vi "DriveStraightCommandNavXRamparts.vi"(6 "TONDelay":u32=50, 8 "speed":dbl=0.8, 9 "Fwd Bwd":dbl, 10 "Delay ms":u32=500, 11 "distance":dbl) -> ()   [LabVIEW 2015]
uses:
  Team Code/Robot Global Data.vi
  NavX/navX Library v2/navX Library v2.lvlib
panel:
  out "isFlat":bool
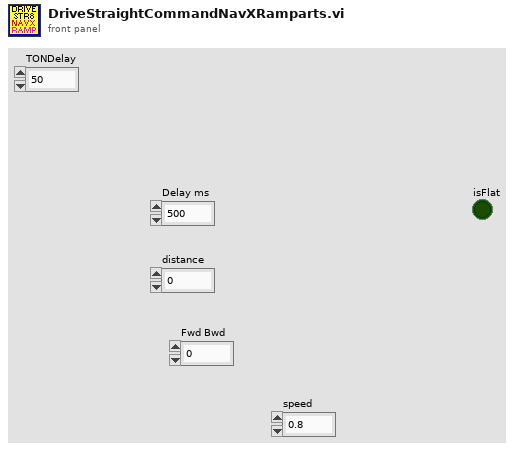
[diagram p1: front panel]
types:
  T1 = enum16{"FlatInitial", "AngleUp", "AngleDown", "FlatFinal"}
  T2 = typedef "WPI_EncoderDevRef.ctl" = cluster{"DevStatus":errorcluster, "EncoderIndex":T3, "CounterIndex":T4, "DistancePerCount":dbl, "Decoding Type":T5}
  T3 = typedef "FPGA_EncoderIdx.ctl" = enum8{"Enc 0", "Enc 1", "Enc 2", "Enc 3", "Enc 4", "Enc 5", "Enc 6", "Enc 7", "Invalid"}
  T4 = typedef "FPGA_CounterCtrSystemIndex.ctl" = enum8{"Ctr 0", "Ctr 1", "Ctr 2", "Ctr 3", "Ctr 4", "Ctr 5", "Ctr 6", "Ctr 7", "Invalid"}
  T5 = typedef "WPI_EncoderType.ctl" = enum16{"1x", "2x", "4x"}
  T6 = typedef "navX Library v2.lvlib/Z900_navX_DeviceTypeDef.ctl" = cluster{"Interface":cluster{"Protocol":T7, "Update Rate (4Hz-60Hz)":u8, "navX Open TypeDef":variant}, "Notify Packet":refnum<notifier>, "Loop VI Refnum":refnum<vi>, "Ready to Close Occurrence Refnum":refnum<k4>}
  T7 = typedef "navX Library v2.lvlib/Z900_navX_ProtocolTypeDef.ctl" = enum16{"SERIAL", "I2C", "SPI"}
  T8 = cluster{"Yaw":dbl, "Roll":dbl, "Pitch":dbl, "Heading":dbl, "Fused Heading":dbl}
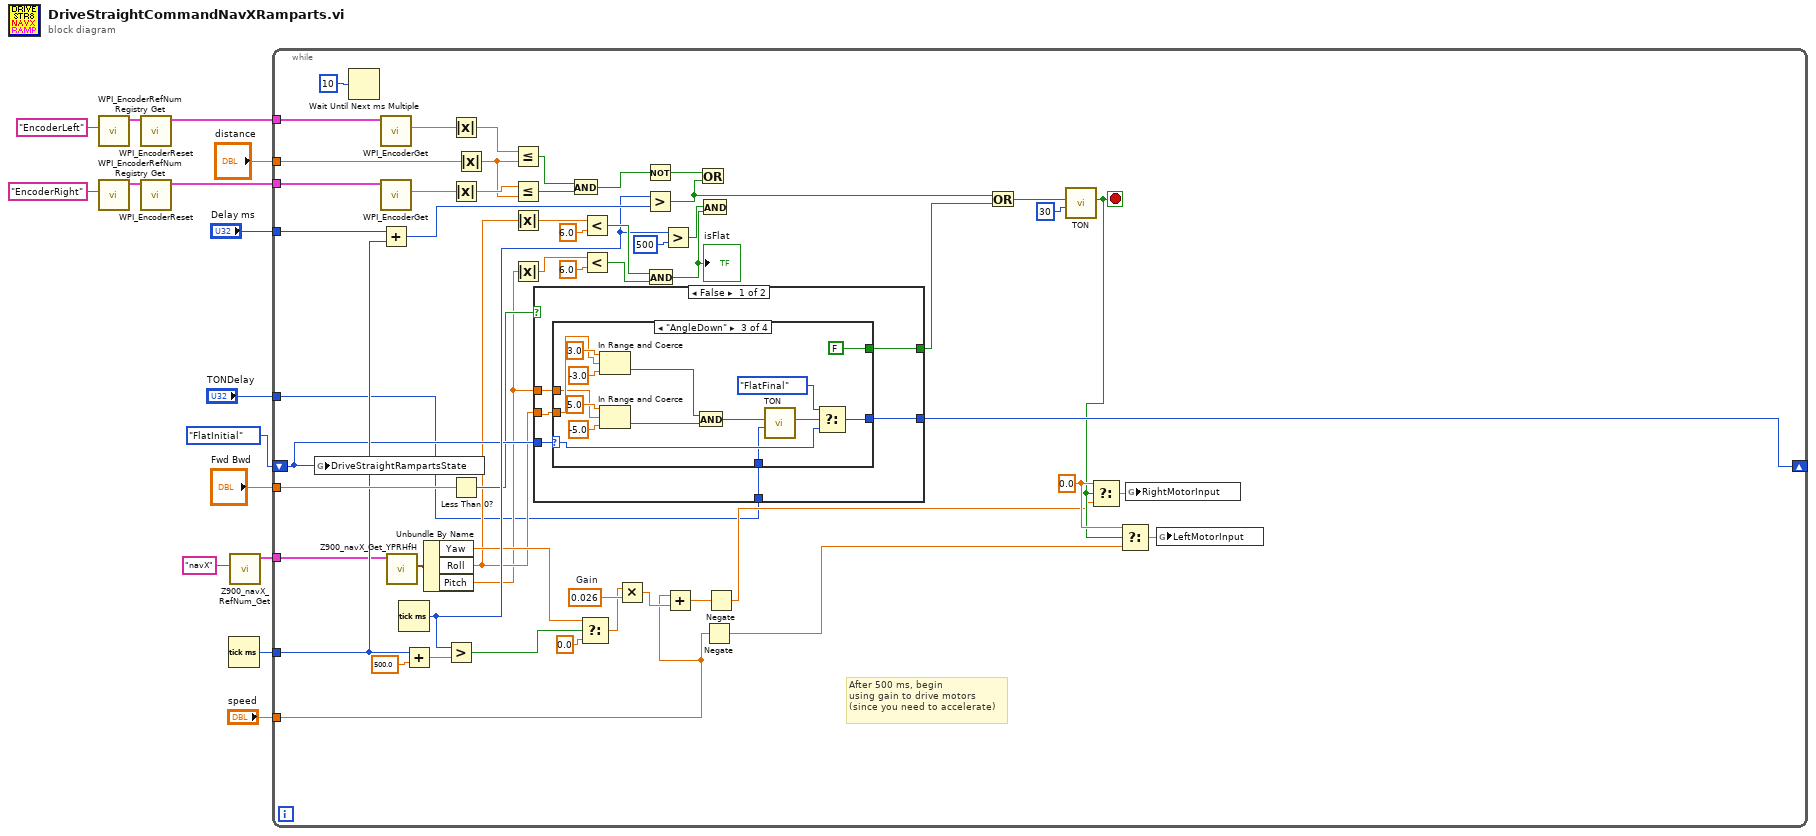
[diagram p0: block diagram]
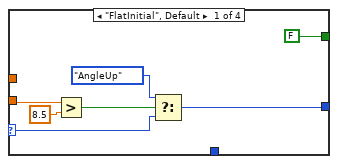
[diagram p2: hidden frame]
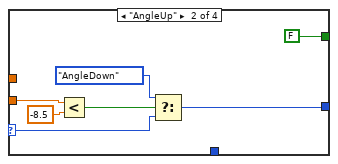
[diagram p3: hidden frame]
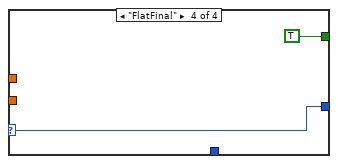
[diagram p4: hidden frame]
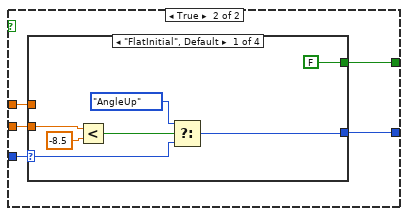
[diagram p5: hidden frame]
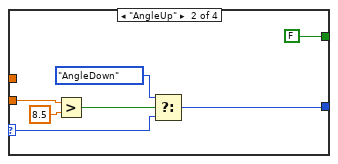
[diagram p6: hidden frame]
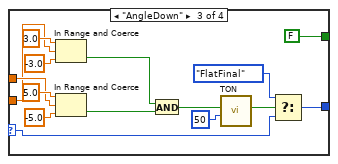
[diagram p7: hidden frame]
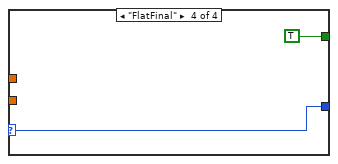
[diagram p8: hidden frame]
diagram:
  n1 = call <vilib>:"WPI_EncoderRefNum Registry Get.vi"("refnum name"="EncoderLeft") -> ("EncoderDevRef"=w14:T2)  [unwired: 9 in, 1 out]
  n2 = call <vilib>:"WPI_EncoderRefNum Registry Get.vi"("refnum name"="EncoderRight") -> ("EncoderDevRef"=w13:T2)  [unwired: 9 in, 1 out]
  n3 = call <vilib>:"WPI_EncoderReset.vi"("EncoderDevRef"=w14) -> ("EncoderDevRef"=w10:T2)  [unwired: 9 in, 1 out]
  n4 = call <vilib>:"WPI_EncoderReset.vi"("EncoderDevRef"=w13) -> ("EncoderDevRef"=w9:T2)  [unwired: 9 in, 1 out]
  n5 = Tick Count (ms)() -> (millisecond timer value=w6:u32)
  n6 = call "Z900_navX_RefNum_Get.vi"("refnum name"="navX") -> ("navX Device"=w4:T6)  [unwired: 9 in, 1 out]
  n7 = while {
    tunnel: "distance" -> [w62]
    tunnel: w10 -> [w65]
    tunnel: w9 -> [w64]
    tunnel: "Fwd Bwd" -> [w63]
    tunnel: "Delay ms" -> [w59]
    tunnel: w6 -> [w57]
    tunnel: w4 -> [w52]
    shift-right: [w40] -> _
    shift-left: T1."FlatInitial" -> [w39]
    tunnel: "speed" -> [w19]
    tunnel: "TONDelay" -> [w16]
    stop <- w18 stop-if-true
    w21 = 0.0 ("t")
    w32 = 0.026  # Gain
    # "After 500 ms, begin\nusing gain to drive motors\n(since you need to accelerate)"
    n8 = global write "Robot Global Data.vi" "DriveStraightRampartsState"(w39) -> ()
    n9 = Wait Until Next ms Multiple(millisecond multiple=u32 10 ("milliseconds to wait")) -> ()  [unwired: 1 out]
    n10 = call <vilib>:"WPI_EncoderGet.vi"("EncoderDevRef"=w65) -> ("Distance"=w66:dbl)  [unwired: 5 in, 5 out]
    n11 = call <vilib>:"WPI_EncoderGet.vi"("EncoderDevRef"=w64) -> ("Distance"=w67:dbl)  [unwired: 5 in, 5 out]
    n12 = Add(x=w59, y=w57) -> (x+y=w60:u32)
    n13 = call "Z900_navX_Get_YPRHfH.vi"("navX Device"=w52) -> ("YRPHfH"=w51:T8)  [unwired: 7 in, 3 out]
    n14 = Tick Count (ms)() -> (millisecond timer value=w44:u32)
    n15 = Add(x=w57, y=500.0) -> (x+y=w56:dbl)
    n16 = Unbundle By Name(w51) -> ("Yaw"=w30:dbl, "Roll"=w26:dbl, "Pitch"=w25:dbl)
    n17 = Greater?(x=w44, y=w56) -> (0:w28:bool)
    n18 = Absolute Value(x=w66) -> (abs(x)=w68:dbl)
    n19 = Absolute Value(x=w67) -> (abs(x)=w70:dbl)
    n20 = Less Than 0?(x=w63) -> (x < 0?=w33:bool)
    n21 = Absolute Value(x=w62) -> (abs(x)=w69:dbl)
    n22 = Less Or Equal?(x=w68, y=w69) -> (x <= y?=w55:bool)
    n23 = Less Or Equal?(x=w70, y=w69) -> (x <= y?=w54:bool)
    n24 = Absolute Value(x=w26) -> (abs(x)=w50:dbl)
    n25 = Absolute Value(x=w25) -> (abs(x)=w47:dbl)
    n26 = case shown="False" w33 {
      tunnel: [w75 w111] -> w40
      tunnel: w39 -> [w74 w112]
      tunnel: [w76 w110] -> w35
      tunnel: w26 -> [w73 w109]
      tunnel: w25 -> [w72 w108]
      tunnel: w16 -> [w71 _]
      frame False {
        n27 = case shown="\"AngleDown\"" w74 {
          selector: w74 -> [w83 w90 w100 w107]
          tunnel: [w81 w88 w101 w107] -> w75
          tunnel: [FALSE FALSE FALSE TRUE] -> w76
          tunnel: w73 -> [w77 w84 w93 _]
          tunnel: w72 -> [_ _ w92 _]
          tunnel: w71 -> [_ _ w91 _]
          frame "FlatInitial", Default {
            n28 = Greater?(x=w77, y=8.5) -> (0:w78:bool)
            n29 = Select(t=T1."AngleUp", s=w78, f=w83) -> (s? t:f=w81:T1)
          }
          frame "AngleUp" {
            n30 = Less?(x=w84, y=-8.5) -> (x < y?=w85:bool)
            n31 = Select(t=T1."AngleDown", s=w85, f=w90) -> (s? t:f=w88:T1)
          }
          frame "AngleDown" {
            n32 = In Range and Coerce(upper limit=3.0, x=w93, lower limit=-3.0) -> (In Range?=w96:bool)  [unwired: 1 out]
            n33 = In Range and Coerce(upper limit=5.0, x=w92, lower limit=-5.0) -> (In Range?=w95:bool)  [unwired: 1 out]
            n34 = And(x=w96, y=w95) -> (x .and. y?=w94:bool)
            n35 = call "TON.vi"("Delay (ms)"=w91, "Input"=w94) -> ("Output"=w99:bool)  [unwired: 9 in]
            n36 = Select(t=T1."FlatFinal", s=w99, f=w100) -> (s? t:f=w101:T1)
          }
          frame "FlatFinal" {
          }
        }
      }
      frame True {
        n37 = case shown="\"FlatInitial\", Default" w112 {
          selector: w112 -> [w119 w126 w136 w143]
          tunnel: [w117 w124 w137 w143] -> w111
          tunnel: [FALSE FALSE FALSE TRUE] -> w110
          tunnel: w109 -> [w113 w120 w127 _]
          tunnel: w108 -> [_ _ w128 _]
          frame "FlatInitial", Default {
            n38 = Less?(x=w113, y=-8.5) -> (x < y?=w114:bool)
            n39 = Select(t=T1."AngleUp", s=w114, f=w119) -> (s? t:f=w117:T1)
          }
          frame "AngleUp" {
            n40 = Greater?(x=w120, y=8.5) -> (0:w121:bool)
            n41 = Select(t=T1."AngleDown", s=w121, f=w126) -> (s? t:f=w124:T1)
          }
          frame "AngleDown" {
            n42 = In Range and Coerce(upper limit=3.0, x=w127, lower limit=-3.0) -> (In Range?=w131:bool)  [unwired: 1 out]
            n43 = In Range and Coerce(upper limit=5.0, x=w128, lower limit=-5.0) -> (In Range?=w130:bool)  [unwired: 1 out]
            n44 = And(x=w131, y=w130) -> (x .and. y?=w129:bool)
            n45 = call "TON.vi"("Delay (ms)"=u32 50, "Input"=w129) -> ("Output"=w135:bool)  [unwired: 9 in]
            n46 = Select(t=T1."FlatFinal", s=w135, f=w136) -> (s? t:f=w137:T1)
          }
          frame "FlatFinal" {
          }
        }
      }
    }
    n47 = And(x=w55, y=w54) -> (x .and. y?=w38:bool)
    n48 = Select(t=w30, s=w28, f=0.0) -> (s? t:f=w29:dbl)
    n49 = Less?(x=w50, y=6.0) -> (x < y?=w48:bool)
    n50 = Less?(x=w47, y=6.0) -> (x < y?=w45:bool)
    n51 = Multiply(x=w29, y=w32) -> (x*y=w31:dbl)
    n52 = Not(x=w38) -> (.not. x?=w53:bool)
    n53 = Greater?(x=w44, y=w60) -> (0:w36:bool)
    n54 = And(x=w48, y=w45) -> (x .and. y?=w41:bool)
    "isFlat" <- w41
    n55 = Greater?(x=w44, y=u32 500) -> (0:w42:bool)
    n56 = Add(x=w19, y=w31) -> (x+y=w20:dbl)
    n57 = Or(x=w53, y=w36) -> ()  [unwired: 1 out]
    n58 = And(x=w42, y=w41) -> ()  [unwired: 1 out]
    n59 = Negate(x=w19) -> (-x=w24:dbl)
    n60 = Negate(x=w20) -> (-x=w17:dbl)
    n61 = Or(x=w36, y=w35) -> (x .or. y?=w34:bool)
    n62 = call "TON.vi"("Delay (ms)"=u32 30, "Input"=w34) -> ("Output"=w18:bool)  [unwired: 9 in]
    n63 = Select(t=w21, s=w18, f=w17) -> (s? t:f=w23:dbl)
    n64 = Select(t=w21, s=w18, f=w24) -> (s? t:f=w22:dbl)
    n65 = global write "Robot Global Data.vi" "RightMotorInput"(w23) -> ()
    n66 = global write "Robot Global Data.vi" "LeftMotorInput"(w22) -> ()
  }
